vi "Actor Core.vi"(8 "error in":errorcluster, 11 "HIJ Multiple Cams App Demo In":refnum<class "HIJ 3 Alignment Cams App.lvclass">) -> (0 "error out":errorcluster, 3 "Actor out":refnum<class "Actor.lvclass">)   [LabVIEW 2014, in "HIJ 3 Alignment Cams App.lvlib" / "HIJ 3 Alignment Cams App.lvclass"]
doc: "(<B>Filename</B>: Actor Framework.lvlib:Actor.lvclass:Actor Core.vi)\n\nReceives messages to the actor, reacts to them, and initiates any error handling that may shut the actor down.\n\nDescendant classes may override this VI to append parallel tasks for the actor to complete while it handles messages. Overrides use the Call Parent Method node."
uses:
  HIJ 3 Alignment Cams App.lvclass
  <vilib>/ActorFramework/Actor/Actor.lvclass
  HIJ Vision App IMAQdx Display/HIJ Vision App IMAQdx Display/HIJ Vision App IMAQdx Display.lvclass
  Analyze/Results and Overlays/Static Text Overlay/Static Text Overlay.lvclass
  Analyze/Results and Overlays/Static Overlay/Static Position.ctl
  Display Actors/HIJ IMAQdx Display/AF IMAQ Display/HIJ IMAQdx Display.lvclass
  Analyze/Results and Overlays/Static Overlay/Static Overlay.lvclass/Static Overlay.ctl
  HIJ 3 Alignment Cams App.lvclass/HIJ 3 Alignment Cams App.ctl
  Display Actors/HIJ Vision Display/HIJ Vision Display/HIJ Vision Display.lvclass/HIJ Vision Display.ctl
  Display Actors/HIJ IMAQdx Display/AF IMAQ Display/HIJ IMAQdx Display.lvclass/HIJ IMAQdx Display.ctl
  HIJ Vision App IMAQdx Display/HIJ Vision App IMAQdx Display/HIJ Vision App IMAQdx Display.lvclass/HIJ Vision App IMAQdx Display.ctl
  Application Base Actors/HIJ Vision Camera App/HIJ Vision Camera App/HIJ Vision Camera App.lvclass/HIJ Vision Camera App.ctl
  CamAppInfo.ctl
  <vilib>/userdefined/High Color/IMAQdx.ctl
  <vilib>/ActorFramework/Message Enqueuer/Message Enqueuer.lvclass
  Analyze/Results and Overlays/Static Text Overlay/Static Text Overlay.lvclass/Static Text Overlay.ctl
  Shared Code/Viewable Actor/ViewableActor Messages/Insert Into SubPanel Msg/Insert Into SubPanel Msg.lvclass/Insert Into SubPanel Msg.ctl
  <vilib>/ActorFramework/Message Enqueuer/Message Enqueuer.lvclass/Message Enqueuer.ctl
  <vilib>/ActorFramework/Actor/Actor.lvclass/Actor.ctl
  HIJ 3 Alignment Cams App Messages/Exchange Main Camera Msg/Exchange Main Camera Msg.lvclass/Exchange Main Camera Msg.ctl
  HIJ 3 Alignment Cams App Messages/Forward Menu Selection Msg/Forward Menu Selection Msg.lvclass/Forward Menu Selection Msg.ctl
  HIJ 3 Alignment Cams App Messages/Menu Activation Msg/Menu Activation Msg.lvclass/Menu Activation Msg.ctl
  Analyze/Results and Overlays/Static Text Overlay/Write OVL Text.vi
  Analyze/Results and Overlays/Static Overlay/Write Static Position.vi
  Display Actors/HIJ Vision Display/HIJ Vision Display/Write WorkDir.vi
  Display Actors/HIJ IMAQdx Display/AF IMAQ Display/Write ConfigDir.vi
  HIJ Vision App IMAQdx Display/HIJ Vision App IMAQdx Display/Write Caller Menu Ref.vi
  Application Base Actors/HIJ Vision Camera App/HIJ Vision Camera App/Write Overlay Font.vi
  <vilib>/ActorFramework/Message Enqueuer/Enqueue.vi
  <vilib>/ActorFramework/Message Enqueuer/Init from Existing Queue.vi
  Application Base Actors/HIJ Vision Camera App/HIJ Vision Camera App/Write my WorkDir.vi
  Application Base Actors/HIJ Vision Camera App/HIJ Vision Camera App/Write my ConfigDir.vi
  Application Base Actors/HIJ Vision Camera App/HIJ Vision Camera App/Write Start Acquisition.vi
  Application Base Actors/HIJ Vision Application/HIJ Vision Application/Write HIJ Vision Display.vi
  Application Base Actors/HIJ Vision Camera App/HIJ Vision Camera App/Write Start Camera.vi
  <vilib>/ActorFramework/Message Priority Queue/Priority Enqueue.vi
  Shared Code/Viewable Actor/ViewableActor Messages/Insert Into SubPanel Msg/Insert Into SubPanel Msg.lvclass
  HIJ 3 Alignment Cams App Messages/Exchange Main Camera Msg/Exchange Main Camera Msg.lvclass
  HIJ 3 Alignment Cams App Messages/Forward Menu Selection Msg/Forward Menu Selection Msg.lvclass
  HIJ 3 Alignment Cams App Messages/Menu Activation Msg/Menu Activation Msg.lvclass
  <vilib>/ActorFramework/Stop Msg/Stop Msg.lvclass
  Shared Code/Viewable Actor/ViewableActor/ViewableActor.lvclass
  Analyze/Results and Overlays/Static Overlay/Static Overlay.lvclass
panel:
  in  "Stop Button":bool
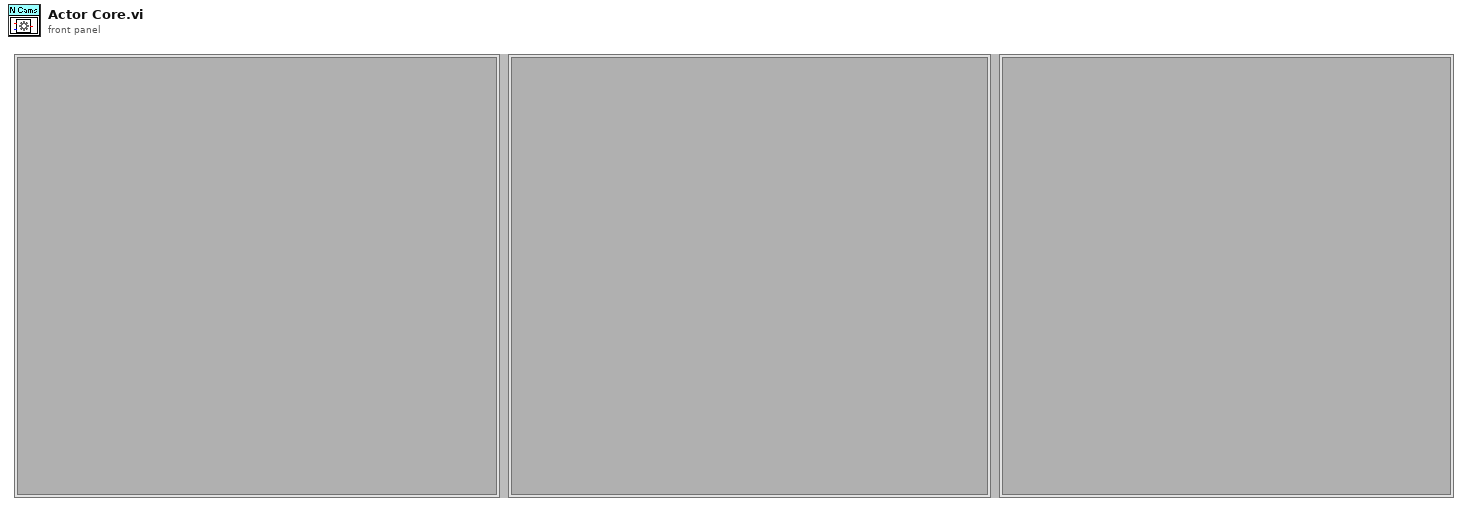
[diagram p1: front panel]
types:
  T1 = cluster{"Desired Font (Application)":enum16{"User-specified Font", "Application Font", "System Font", "Dialog Font"}, "[User-specified Font]":cluster{"Font Name":string, "Size":i16, "Strikeout?":bool, "Italic?":bool, "Underline?":bool, "Outline?":bool, "Shadow?":bool, "Bold?":bool, "Rotation Angle":dbl}, "Horizontal Alignment":i16, "Vertical Alignment":i16}
  T2 = typedef "Static Overlay.lvclass/Static Position.ctl" = enum16{"Top Left", "Top Center", "Top Right", "Center", "Bottom Left", "Bottom Center", "Bottom Right"}
  T3 = typedef "IMAQdx.ctl" = refnum<k21>
  T4 = typedef "HIJ 3 Alignment Cams App.lvlib/HIJ 3 Alignment Cams App.lvclass/CamAppInfo.ctl" = cluster{"Camera":T3, "App enq":refnum<class "Message Enqueuer.lvclass">, "SubPnl Refnum":refnum<vi>}
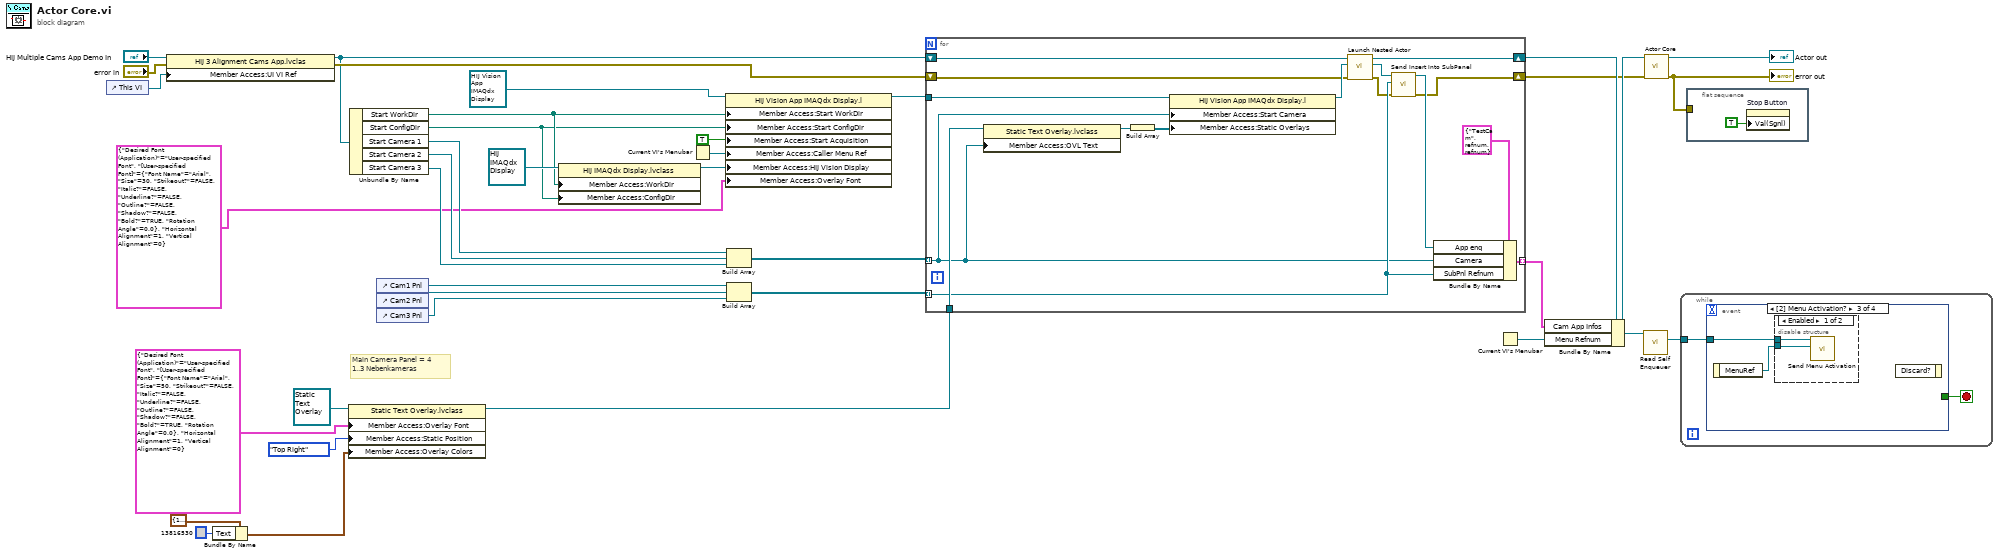
[diagram p0: block diagram]
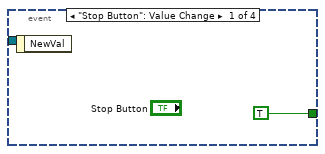
[diagram p2: hidden frame]
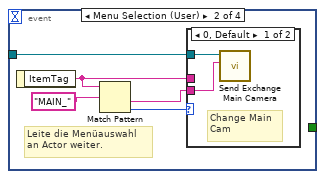
[diagram p3: hidden frame]
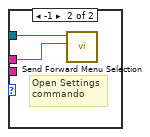
[diagram p4: hidden frame]
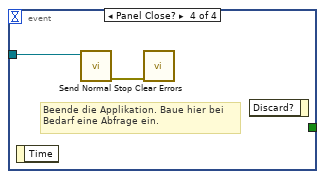
[diagram p6: hidden frame]
diagram:
  # "Main Camera Panel = 4\n1..3 Nebenkameras"
  n1 = control-ref of="This VI"() -> (w32:refnum<vi>)
  n2 = property class="HIJ 3 Alignment Cams App.lvclas"(reference="HIJ Multiple Cams App Demo In", error in="error in", "Member Access:UI VI Ref"=w32) -> (reference out=w28:refnum<class "HIJ 3 Alignment Cams App.lvclass">, error out=w30:errorcluster)
  n3 = Bundle By Name(cluster=cluster{"Border":u32, "Text":u32} {"Border"=16448250, "Text"=16448250} ("Overlay Colors"), "Text"=u32 13816530) -> (w8:cluster{"Border":u32, "Text":u32})
  n4 = property class="Static Text Overlay.lvclass"(reference=refnum<class "Static Text Overlay.lvclass"> refnum ("Static Text Overlay.lvclass"), "Member Access:Overlay Font"=T1 {"Desired Font (Application)"=enum."User-specified Font", "[User-specified Font]"={"Font Name"="Arial", "Size"=50, "Strikeout?"=FALSE, "Italic?"=FALSE, "Underline?"=FALSE, "Outline?"=FALSE, "Shadow?"=FALSE, "Bold?"=TRUE, "Rotation Angle"=0.0}, "Horizontal Alignment"=1, "Vertical Alignment"=0} ("Overlay Font"), "Member Access:Static Position"=Static_Position."Top Right" ("Static Position"), "Member Access:Overlay Colors"=w8) -> (reference out=w11:refnum<class "Static Text Overlay.lvclass">)  [unwired: 1 in, 1 out]
  n5 = Unbundle By Name(w28) -> ("Start WorkDir"=w5:path, "Start ConfigDir"=w4:path, "Start Camera 1"=w25:T3, "Start Camera 2"=w24:T3, "Start Camera 3"=w23:T3)
  n6 = control-ref of="Cam1 Pnl"() -> (w20:refnum<vi>)
  n7 = control-ref of="Cam2 Pnl"() -> (w19:refnum<vi>)
  n8 = control-ref of="Cam3 Pnl"() -> (w18:refnum<vi>)
  n9 = property class="HIJ IMAQdx Display.lvclass"(reference=refnum<class "HIJ IMAQdx Display.lvclass"> refnum ("HIJ IMAQdx Display.lvlib:HIJ IMAQdx Display.lvclass"), "Member Access:WorkDir"=w5, "Member Access:ConfigDir"=w4) -> (reference out=w3:refnum<class "HIJ IMAQdx Display.lvclass">)  [unwired: 1 in, 1 out]
  n10 = Current VI's Menubar() -> (w27:refnum<k9>)
  n11 = property class="HIJ Vision App IMAQdx Display.l"(reference=refnum<class "HIJ Vision App IMAQdx Display.lvclass"> refnum ("HIJ Vision App IMAQdx Display.lvlib:HIJ Vision App IMAQdx Display.lvclass"), "Member Access:Start WorkDir"=w5, "Member Access:Start ConfigDir"=w4, "Member Access:Start Acquisition"=TRUE ("Start Acquisition"), "Member Access:Caller Menu Ref"=w27, "Member Access:HIJ Vision Display"=w3, "Member Access:Overlay Font"=T1 {"Desired Font (Application)"=enum."User-specified Font", "[User-specified Font]"={"Font Name"="Arial", "Size"=30, "Strikeout?"=FALSE, "Italic?"=FALSE, "Underline?"=FALSE, "Outline?"=FALSE, "Shadow?"=FALSE, "Bold?"=TRUE, "Rotation Angle"=0.0}, "Horizontal Alignment"=1, "Vertical Alignment"=0} ("Overlay Font")) -> (reference out=w26:refnum<class "HIJ Vision App IMAQdx Display.lvclass">)  [unwired: 1 in, 1 out]
  n12 = Build Array(w25, w24, w23) -> (w13:T3[])
  n13 = Build Array(w20, w19, w18) -> (w17:refnum<vi>[])
  n14 = for {
    tunnel: w26 -> [w39]
    shift-right: [w44] -> w21
    shift-left: w30 -> [w49]
    shift-right: [w47] -> w29
    shift-left: w28 -> [w45]
    tunnel: w17 -> [w50] mode=indexing
    tunnel: w13 -> [w41] mode=indexing
    tunnel: [w43] -> w16 mode=indexing
    tunnel: w11 -> [w53]
    n15 = property class="Static Text Overlay.lvclass"(reference=w53, "Member Access:OVL Text"=w41) -> (reference out=w40:refnum<class "Static Text Overlay.lvclass">)  [unwired: 1 in, 1 out]
    n16 = Build Array(w40) -> (w38:refnum<class "Static Text Overlay.lvclass">[])
    n17 = property class="HIJ Vision App IMAQdx Display.l"(reference=w39, "Member Access:Start Camera"=w41, "Member Access:Static Overlays"=w38) -> (reference out=w52:refnum<class "HIJ Vision App IMAQdx Display.lvclass">)  [unwired: 1 in, 1 out]
    n18 = call <vilib>:"Launch Nested Actor.vi"("error in (no error)"=w49, "Nested Actor"=w52, "Caller Actor in"=w45) -> ("error out"=w46:errorcluster, "Nested Actor's Enqueuer"=w48:refnum<class "Message Enqueuer.lvclass">, "Caller Actor out"=w47:refnum<class "HIJ 3 Alignment Cams App.lvclass">)  [unwired: 6 in]
    n19 = call "Send Insert Into SubPanel.vi"("error in (no error)"=w46, "SubPanel Ref"=w50, "Message Enqueuer"=w48) -> ("error out"=w44:errorcluster, "Message Enqueuer out"=w51:refnum<class "Message Enqueuer.lvclass">)  [unwired: 7 in]
    n20 = Bundle By Name(cluster=T4 {"Camera"="TestCam", "App enq"=refnum, "SubPnl Refnum"=refnum} ("Cam app info"), "App enq"=w51, "Camera"=w41, "SubPnl Refnum"=w50) -> (w43:T4)
  }
  n21 = Current VI's Menubar() -> (w14:refnum<k9>)
  n22 = Bundle By Name(cluster=w29, "Cam App Infos"=w16, "Menu Refnum"=w14) -> (w22:refnum<class "HIJ 3 Alignment Cams App.lvclass">)
  n23 = call <vilib>:"Read Self Enqueuer.vi"("Actor"=w22) -> ("Self Enqueuer"=w35:refnum<class "Message Enqueuer.lvclass">)  [unwired: 10 in]
  n24 = call-parent "Actor Core.vi"("error in"=w21, "Actor in"=w22) -> ("error out"=w36:errorcluster, "Actor out"=→"Actor out":refnum<class "Actor.lvclass">)  [unwired: 8 in]
  "error out" <- w36
  n25 = while {
    tunnel: w35 -> [w54]
    stop <- w55 stop-if-true
    n26 = event shown="[2] Menu Activation?" {
      selector: _ -> [_ _ _ _]
      dyn-events: _ -> [_ _ _ _]
      timeout: _ -> [_ _ _ _]
      tunnel: [TRUE _ _ _] -> w55
      tunnel: w54 -> [_ w61 w67 w71]
      event "Stop Button": Value Change {
        n27 = event-data() -> ()  [unwired: 1 in, 1 out]
      }
      event Menu Selection (User) {
        # "Leite die Menüauswahl \nan Actor weiter."
        n28 = event-data() -> ("ItemTag"=w60:string)  [unwired: 1 in]
        n29 = Match Pattern(string=w60, regular expression="MAIN_" ("menu tag")) -> (after substring=w57:string, offset past match=w58:i32)  [unwired: 1 in, 2 out]
        n30 = case shown="0, Default" w58 {
          tunnel: w61 -> [w63 w65]
          tunnel: w60 -> [_ w64]
          tunnel: w57 -> [w62 _]
          frame 0, Default {
            # "Change Main\nCam"
            n31 = call "Send Exchange Main Camera.vi"("New Main Cam"=w62, "Message Enqueuer"=w63) -> ()  [unwired: 8 in, 2 out]
          }
          frame -1 {
            # "Open Settings\ncommando"
            n32 = call "Send Forward Menu Selection.vi"("MenuTag"=w64, "Message Enqueuer"=w65) -> ()  [unwired: 8 in, 2 out]
          }
        }
      }
      event Menu Activation? {
        n33 = event-data() -> ("MenuRef"=w66:refnum<k9>)  [unwired: 1 in]
        n34 = disable-structure shown="Enabled" {
          disable-tunnel: w67 -> [w69 _]
          disable-tunnel: w66 -> [w68 _]
          frame Enabled {
            n35 = call "Send Menu Activation.vi"("Menu Refnum"=w68, "Message Enqueuer"=w69) -> ()  [unwired: 8 in, 2 out]
          }
          frame Disabled {
          }
        }
        n36 = event-data() -> ()  [unwired: 2 in, 1 out]
      }
      event Panel Close? {
        # "Beende die Applikation. Baue hier bei\nBedarf eine Abfrage ein."
        n37 = event-data() -> ()  [unwired: 1 in, 1 out]
        n38 = call <vilib>:"Send Normal Stop.vi"("Message Enqueuer"=w71) -> ("error out"=w70:errorcluster)  [unwired: 10 in]
        n39 = call <vilib>:"Clear Errors.vi"("error in (no error)"=w70) -> ()  [unwired: 5 in, 2 out]
        n40 = event-data() -> ()  [unwired: 2 in, 1 out]
      }
    }
  }
  n41 = flat-sequence {
    tunnel: w36 -> [_]
    frame #0 {
      n42 = property on="Stop Button" class="Bool (strict)"("Val(Sgnl)"=TRUE) -> ()  [unwired: 2 in, 2 out]
    }
  }
